vi "whitenoise_v0.vi"(8 "error in (no error)":errorcluster) -> (0 "error out":errorcluster)   [LabVIEW 2017]
uses:
  <vilib>/sound2/lvsound2.llb/Sound Data Format.ctl
  <vilib>/sound2/lvsound2.llb/Sampling Mode.ctl
  Global_InitEndSync.vi
  <vilib>/sound2/lvsound2.llb/Sound Output Set Volume (Single).vi
  <vilib>/sound2/lvsound2.llb/Sound Output Write (DBL Single).vi
  <vilib>/measure/NI_MABase.lvlib
panel:
  in  "Volume":dbl(knob)=100.0 scale=0.0..100.0
  in  "stop":bool
  in  "Time limit (ms)":dbl=inf
  in  "Sound Format":T1={"sample rate (S/s)"=96000.0, "number of channels"=2, "bits per sample"=16} caption="サウンド形式"
  in  "Number of Samples/ch":i32=5000 caption="サンプル数/CH"
  in  "Device ID":u32 caption="デバイスID"
  in  "Frequency":dbl=1000.0 caption="周波数" format="%0.2p"
  in  "Waveform Type":T2(ring)=enum."WN" caption="波形タイプ"
  out "Generated Sound":waveform(dbl)(graph) caption="生成されたサウンド"
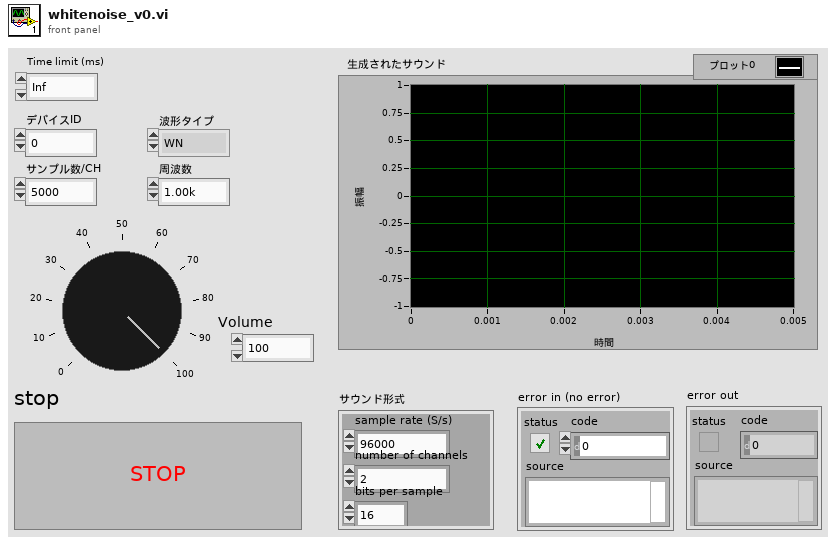
[diagram p1: front panel]
types:
  T1 = typedef "Sound Data Format.ctl" = cluster{"sample rate (S/s)":dbl, "number of channels":i32, "bits per sample":i32}
  T2 = enum16{"Sine", "Square", "WN", "Sawtooth", "Triangle"}
  T3 = typedef "Sampling Mode.ctl" = i32
  T4 = typedef "Sound Output Task ID.ctl" = u32
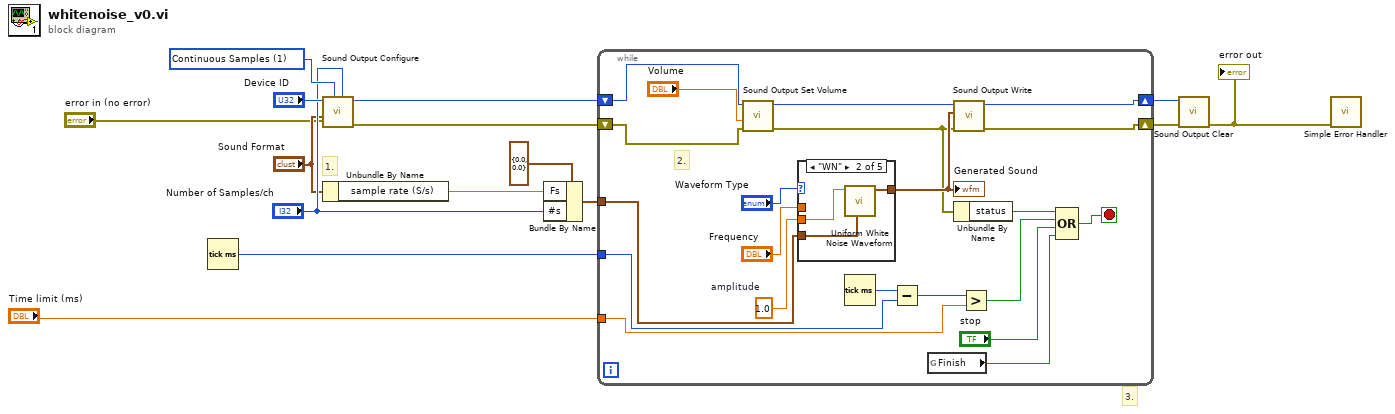
[diagram p0: block diagram]
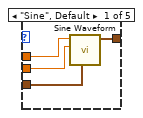
[diagram p2: hidden frame]
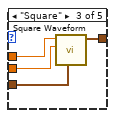
[diagram p3: hidden frame]
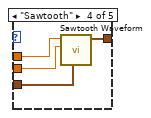
[diagram p4: hidden frame]
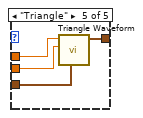
[diagram p5: hidden frame]
diagram:
  w10 = T3 1 items=["Finite Samples", "Continuous Samples"] ("sample mode")
  # "3."
  # "1."
  n1 = Tick Count (ms)() -> (millisecond timer value=w3:u32)
  n2 = call <vilib>:"Sound Output Configure.vi"("number of samples/ch"="Number of Samples/ch", "sample mode"=w10, "error in (no error)"="error in (no error)", "sound format"="Sound Format", "device ID"="Device ID") -> ("error out"=w15:errorcluster, "task ID"=w14:T4)  [unwired: 5 in]
  n3 = Unbundle By Name("Sound Format") -> ("sample rate (S/s)"=w5:dbl)
  n4 = Bundle By Name(cluster=cluster{"Fs":dbl, "#s":dbl} {"Fs"=0.0, "#s"=0.0} ("sampling info"), "Fs"=w5, "#s"="Number of Samples/ch") -> (w7:cluster{"Fs":dbl, "#s":dbl})
  n5 = while {
    shift-right: [w35] -> w13
    shift-left: w15 -> [w26]
    shift-right: [w36] -> w12
    shift-left: w14 -> [w24]
    tunnel: w7 -> [w31]
    tunnel: w3 -> [w22]
    tunnel: "Time limit (ms)" -> [w20]
    stop <- w34 stop-if-true
    w29 = 1.0  # amplitude
    # "2."
    n6 = call-poly <vilib>:"Sound Output Set Volume.vi"("error in (no error)"=w26, "volume"="Volume", "task ID"=w24) -> ("error out"=w27:errorcluster, "task ID out"=w25:T4)  [unwired: 7 in]
    n7 = case shown="\"WN\"" "Waveform Type" {
      tunnel: "Frequency" -> [w40 _ w46 w48 w55]
      tunnel: [w39 w41 w45 w50 w54] -> w28
      tunnel: w31 -> [w38 w43 w47 w51 w53]
      tunnel: w29 -> [w37 w42 w44 w49 w52]
      frame "Sine", Default {
        n8 = call <vilib>:"Sine Waveform.vi"("sampling info"=w38, "amplitude"=w37, "frequency"=w40) -> ("signal out"=w39:waveform(dbl))  [unwired: 7 in, 1 out]
      }
      frame "WN" {
        n9 = call <vilib>:"Uniform White Noise Waveform.vi"("sampling info"=w43, "amplitude"=w42) -> ("signal out"=w41:waveform(dbl))  [unwired: 8 in, 1 out]
      }
      frame "Square" {
        n10 = call <vilib>:"Square Waveform.vi"("sampling info"=w47, "amplitude"=w44, "frequency"=w46) -> ("signal out"=w45:waveform(dbl))  [unwired: 7 in, 1 out]
      }
      frame "Sawtooth" {
        n11 = call <vilib>:"Sawtooth Waveform.vi"("sampling info"=w51, "amplitude"=w49, "frequency"=w48) -> ("signal out"=w50:waveform(dbl))  [unwired: 7 in, 1 out]
      }
      frame "Triangle" {
        n12 = call <vilib>:"Triangle Waveform.vi"("sampling info"=w53, "amplitude"=w52, "frequency"=w55) -> ("signal out"=w54:waveform(dbl))  [unwired: 7 in, 1 out]
      }
    }
    "Generated Sound" <- w28
    n13 = Tick Count (ms)() -> (millisecond timer value=w23:u32)
    n14 = Subtract(x=w23, y=w22) -> (x-y=w21:u32)
    n15 = global read "Global_InitEndSync.vi" "Finish"() -> (w16:bool)
    n16 = call-poly <vilib>:"Sound Output Write.vi"("error in (no error)"=w27, "data"=w28, "task ID"=w25) -> ("error out"=w35:errorcluster, "task ID out"=w36:T4)  [unwired: 7 in]
    n17 = Unbundle By Name(w27) -> ("status"=w32:bool)
    n18 = Greater?(x=w21, y=w20) -> (0:w19:bool)
    n19 = Compound Arithmetic op=OR(w32, w19, "stop", w16) -> (w34:bool)
  }
  n20 = call <vilib>:"Sound Output Clear.vi"("error in (no error)"=w13, "task ID"=w12) -> ("error out"=w6:errorcluster)  [unwired: 9 in]
  "error out" <- w6
  n21 = call <vilib>:"Simple Error Handler.vi"("error in (no error)"=w6) -> ()  [unwired: 4 in, 5 out]
